vi "Main.vi"() -> ()   [LabVIEW 2017]
doc: "Main Vi para Jogo da Velha Multiplayer - Player x Player na mesma máquina, Player x Player pela rede, Player x Computador"
uses:
  controls/Tabuleiro.ctl
  controls/DataOut.ctl
  controls/GameOption.ctl
  controls/DataIn.ctl
  controls/States.ctl
  controls/LogStates.ctl
  controls/TabuleiroCoordenadas.ctl
panel:
  in  "Reiniciar":bool
  in  "Sair":bool
  out "DataOut":T1
  out "Quem joga":string
  out "Tabuleiro":T2
  # "JOGO DA VELHA"
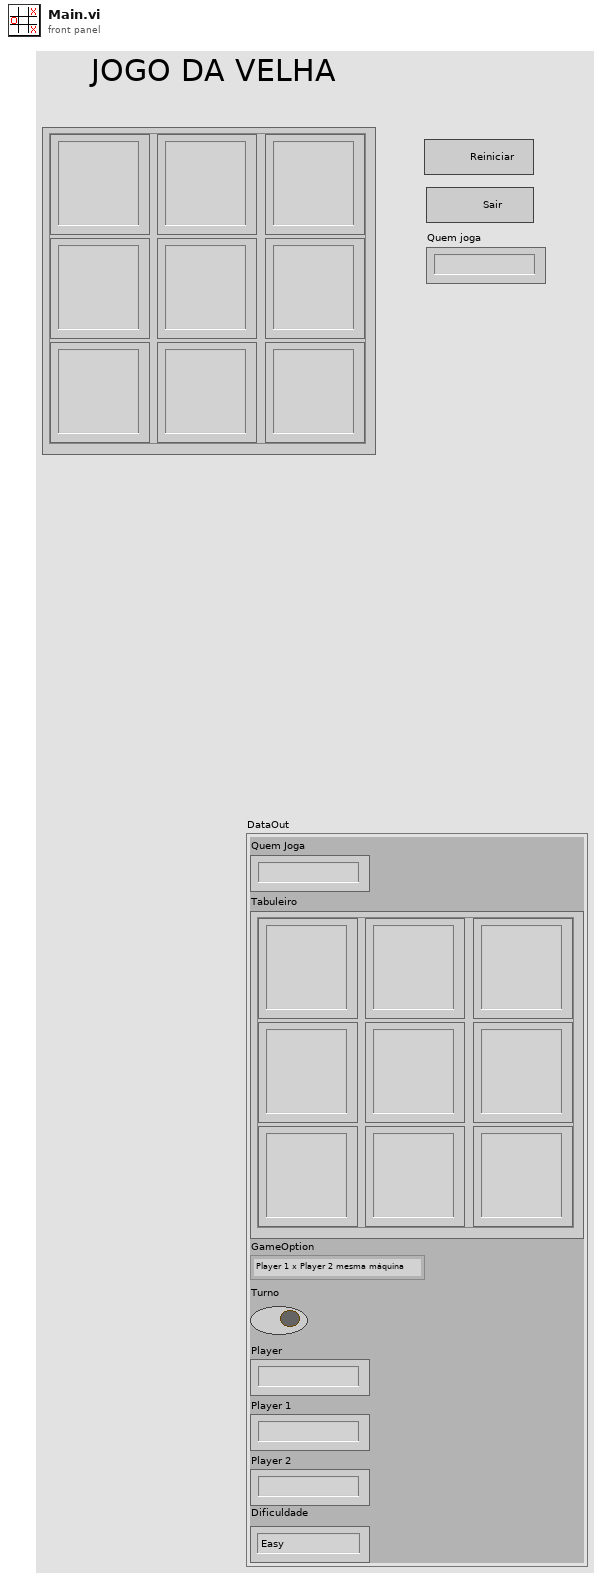
[diagram p1: front panel]
types:
  T1 = typedef "DataOut.ctl" = cluster{"Quem Joga":string, "Tabuleiro":T2, "GameOption":T3, "Turno":bool, "Player":string, "Player 1":string, "Player 2":string, "Dificuldade":enum16{"Easy", "Medium", "Hard"}}
  T2 = typedef "Tabuleiro.ctl" = cluster{"(0,0)":string, "(1,0)":string, "(0,1)":string, "(1,1)":string, "(2,0)":string, "(1,2)":string, "(2,2)":string, "(0,2)":string, "(2,1) ":string}
  T3 = typedef "GameOption.ctl" = enum16{"Player 1 x Player 2 mesma máquina", "Player 1 x Player 2 pela rede", "Player 1 x Computador", "Wait for Event", "Initialize", "Stop"}
  T4 = typedef "States.ctl" = enum16{"Initialize", "Player (wait for event)", "Stop", "PC", "Restart"}
  T5 = typedef "DataIn.ctl" = cluster{"Quem Joga":string, "Tabuleiro":T2, "GameOption":T3, "Turno":bool, "Player":string, "Player 1":string, "Player 2":string, "Dificuldade":enum16{"Easy", "Medium", "Hard"}}
  T6 = typedef "LogStates.ctl" = enum16{"Initialize", "Write", "Write (win, draw)", "Write (PC first)", "Write (Player first)", "Close"}
  T7 = typedef "TabuleiroCoordenadas.ctl" = enum16{"0,0", "0,1", "0,2", "1,0", "1,1", "1,2", "2,0", "2,1", "2,2"}
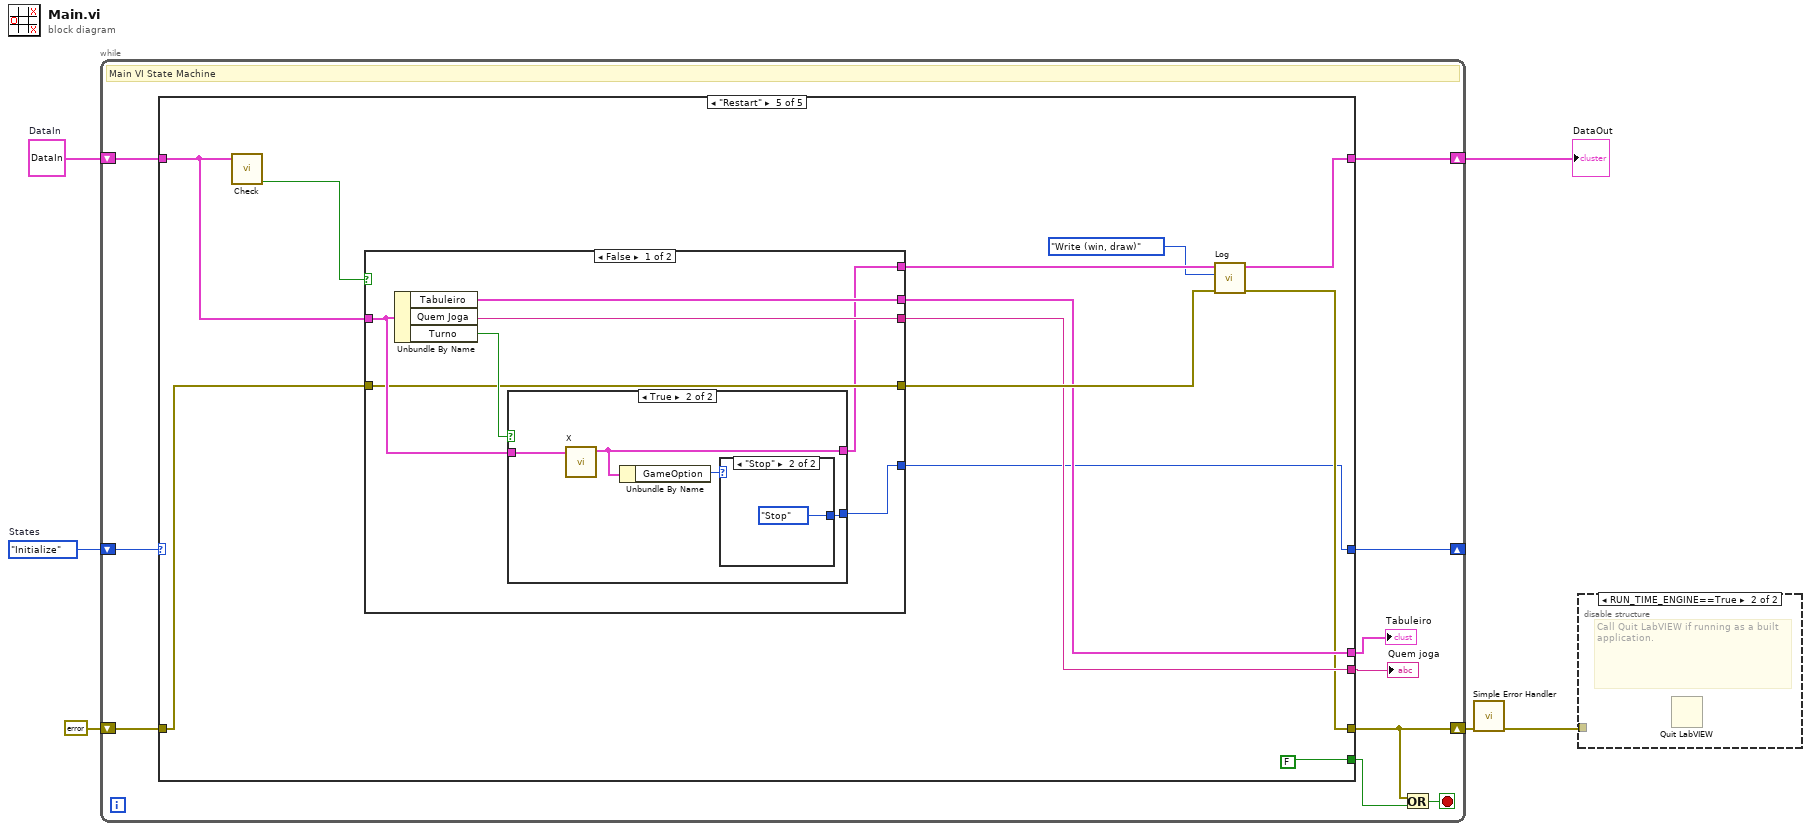
[diagram p0: block diagram]
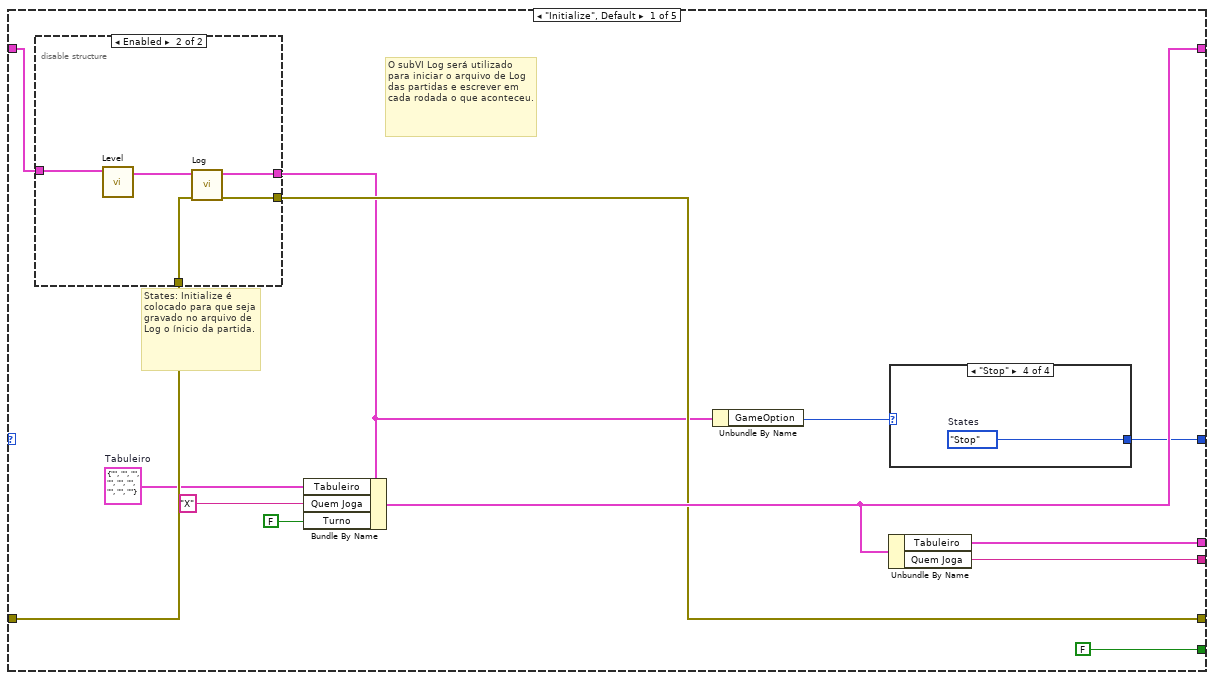
[diagram p2: hidden frame]
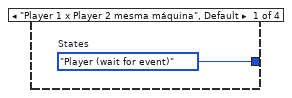
[diagram p3: hidden frame]
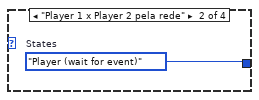
[diagram p4: hidden frame]
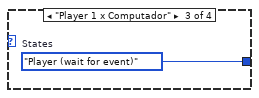
[diagram p5: hidden frame]
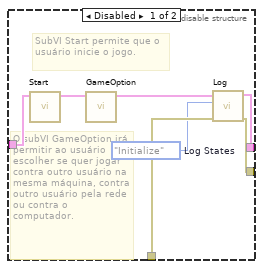
[diagram p6: hidden frame]
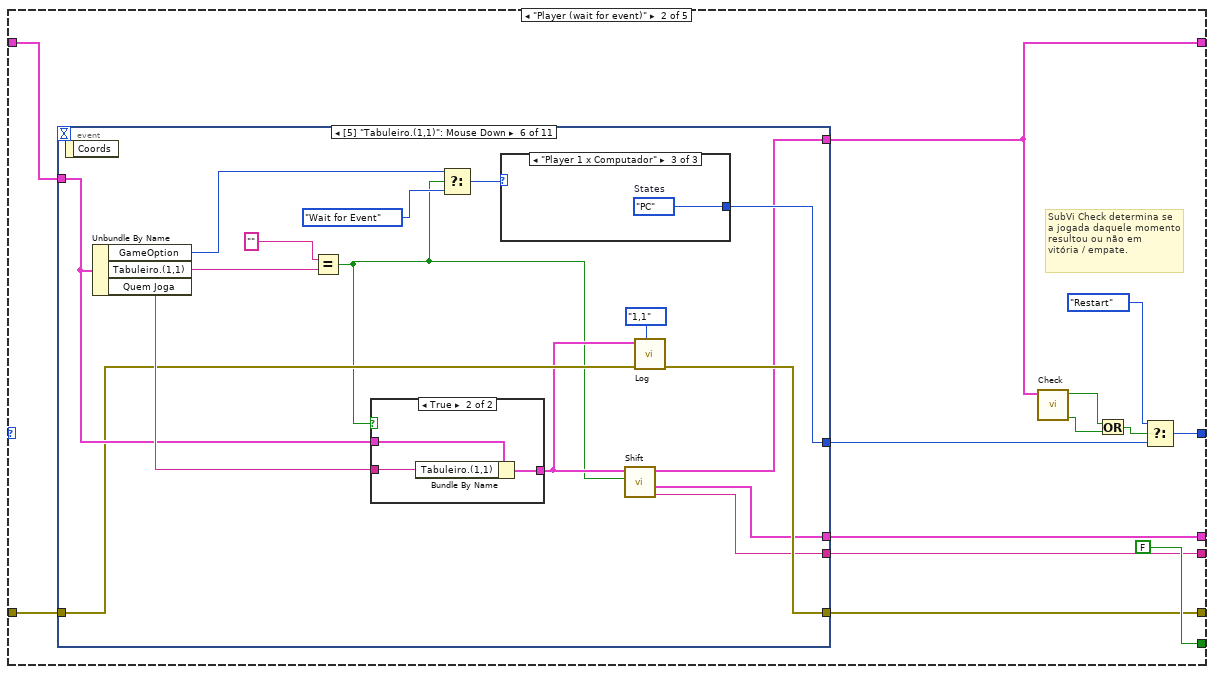
[diagram p7: hidden frame]
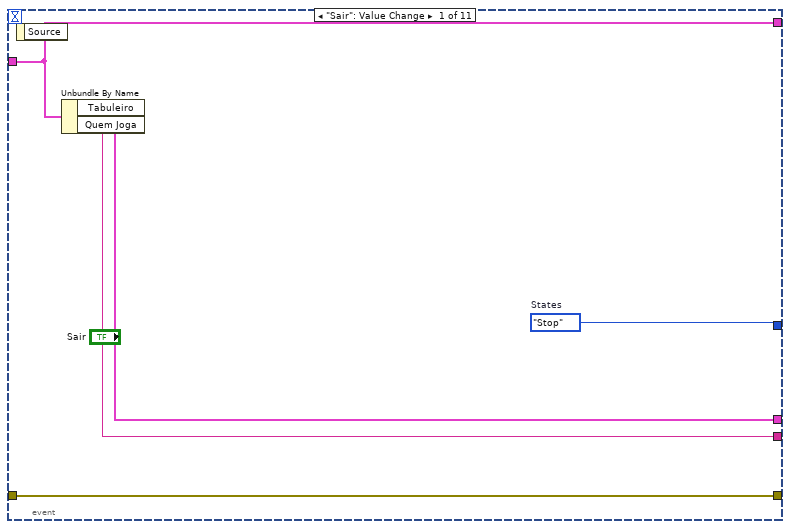
[diagram p8: hidden frame]
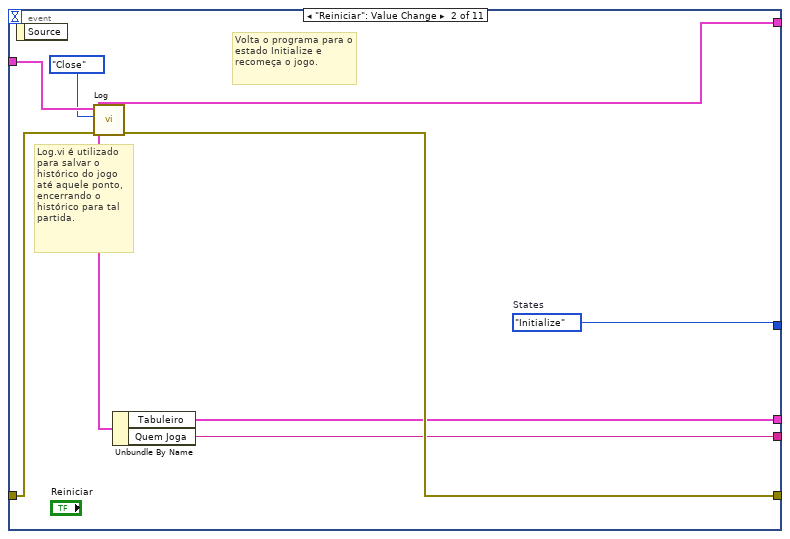
[diagram p9: hidden frame]
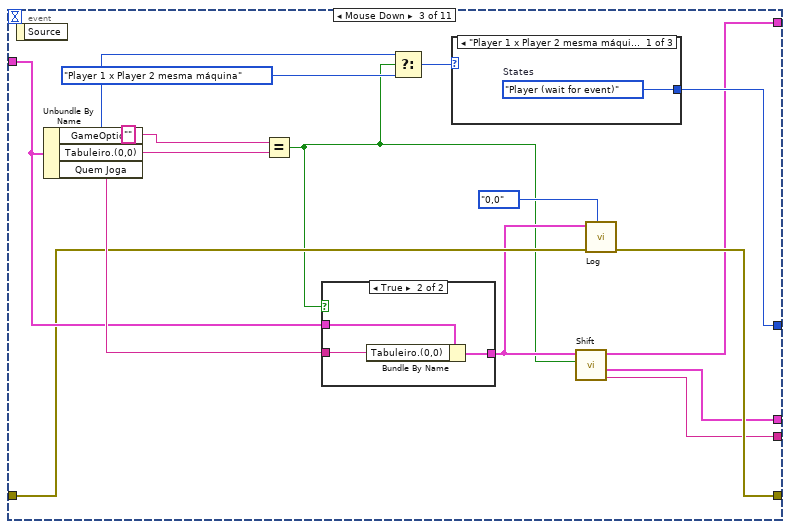
[diagram p10: hidden frame]
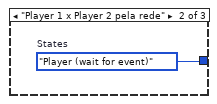
[diagram p12: hidden frame]
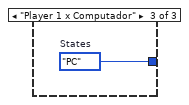
[diagram p13: hidden frame]
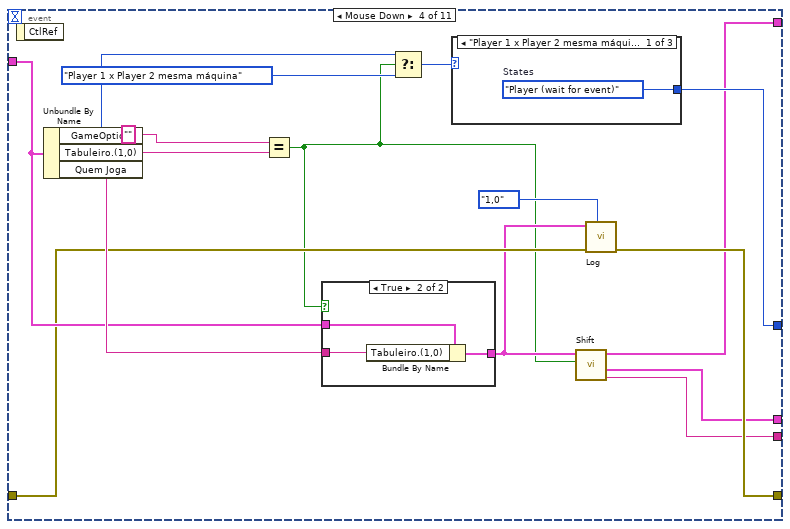
[diagram p14: hidden frame]
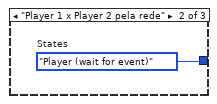
[diagram p16: hidden frame]
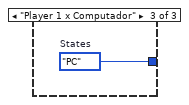
[diagram p17: hidden frame]
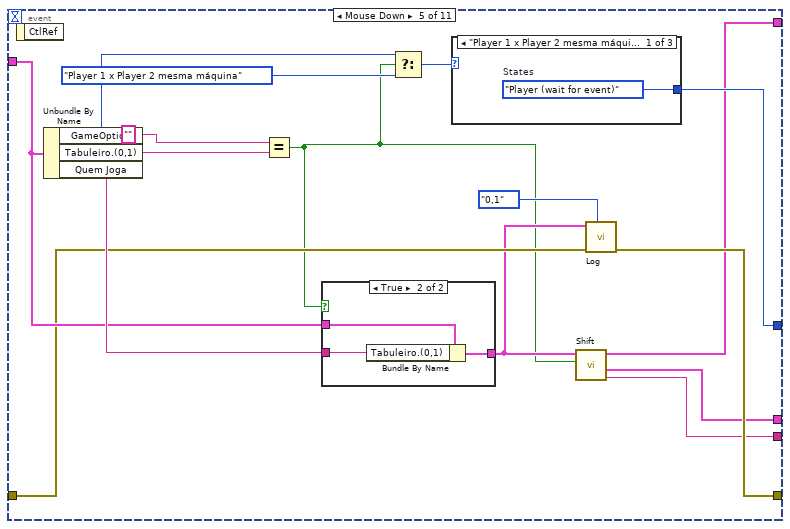
[diagram p18: hidden frame]
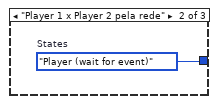
[diagram p20: hidden frame]
diagram:
  w2 = States."Initialize"  # States
  w3 = T5 {"Quem Joga"="", "Tabuleiro"={"(0,0)"="", "(1,0)"="", "(0,1)"="", "(1,1)"="", "(2,0)"="", "(1,2)"="", "(2,2)"="", "(0,2)"="", "(2,1) "=""}, "GameOption"=enum."Player 1 x Player 2 mesma máquina", "Turno"=FALSE, "Player"="", "Player 1"="", "Player 2"="", "Dificuldade"=enum."Easy"}  # DataIn
  n1 = while {
    shift-right: [w13] -> w1
    shift-left: w3 -> [w14]
    shift-right: [w11] -> w5
    shift-left: errorcluster {"status"=FALSE, "code"=0, "source"=""} ("error constant") -> [w12]
    shift-right: [w10] -> _
    shift-left: w2 -> [w15]
    stop <- w16 stop-if-true
    # "Main VI State Machine"
    n2 = case shown="\"Restart\"" w15 {
      tunnel: w14 -> [w28 w57 w282 w286 w313]
      tunnel: [w24 w46 w282 w285 w305] -> w13
      tunnel: w12 -> [w29 w56 w284 w288 w312]
      tunnel: [w20 w55 w284 w288 w306] -> w11
      tunnel: [w17 w51 w283 w291 w304] -> w10
      tunnel: [w23 w54 w281 w290 w310] -> w9
      tunnel: [w22 w53 w280 w289 w309] -> w8
      tunnel: [FALSE FALSE TRUE FALSE FALSE] -> w7
      frame "Initialize", Default {
        w25 = T2 {"(0,0)"="", "(1,0)"="", "(0,1)"="", "(1,1)"="", "(2,0)"="", "(1,2)"="", "(2,2)"="", "(0,2)"="", "(2,1) "=""}  # Tabuleiro
        # "States: Initialize é colocado para que seja gravado no arquivo de Log o ínicio da partida."
        # "O subVI Log será utilizado para iniciar o arquivo de Log das partidas e escrever em cada rodada o que aconteceu."
        n3 = disable-structure shown="Enabled" {
          disable-tunnel: w29 -> [w40 w43]
          disable-tunnel: w28 -> [w39 w41]
          disable-tunnel: [w38 w45] -> w19
          disable-tunnel: [w36 w44] -> w20
          frame Disabled {
            w37 = LogStates."Initialize"  # Log States
            # "SubVI Start permite que o usuário inicie o jogo."
            # "O subVI GameOption irá permitir ao usuário escolher se quer jogar contra outro usuário na mesma máquina, contra outro usuário pela rede ou contra o computador."
            n4 = call "Start.vi"("DataIn"=w39) -> ("Cluster"=w35:T1)  [unwired: 10 in]
            n5 = call "GameOption.vi"("DataIn"=w35) -> ("DataOut"=w34:T1)  [unwired: 10 in]
            n6 = call "Log.vi"("Error In"=w40, "Log States"=w37, "DataIn"=w34) -> ("Error Out"=w36:errorcluster, "DataOut"=w38:T1)  [unwired: 7 in]
          }
          frame Enabled {
            n7 = call "Level.vi"("DataIn"=w41) -> ("Cluster"=w42:T1)  [unwired: 10 in]
            n8 = call "Log.vi"("Error In"=w43, "DataIn"=w42) -> ("Error Out"=w44:errorcluster, "DataOut"=w45:T1)  [unwired: 8 in]
          }
        }
        n9 = Bundle By Name(cluster=w19, "Tabuleiro"=w25, "Quem Joga"="X", "Turno"=FALSE) -> (w24:T1)
        n10 = Unbundle By Name(w19) -> ("GameOption"=w18:T3)
        n11 = Unbundle By Name(w24) -> ("Tabuleiro"=w22:T2, "Quem Joga"=w23:string)
        n12 = case shown="\"Stop\"" w18 {
          tunnel: [w30 w31 w32 w33] -> w17
          frame "Player 1 x Player 2 mesma máquina", Default {
            w30 = States."Player (wait for event)"  # States
          }
          frame "Player 1 x Player 2 pela rede" {
            w31 = States."Player (wait for event)"  # States
          }
          frame "Player 1 x Computador" {
            w32 = States."Player (wait for event)"  # States
          }
          frame "Stop" {
            w33 = States."Stop"  # States
          }
        }
      }
      frame "Player (wait for event)" {
        # "SubVi Check determina se a jogada daquele momento resultou ou não em vitória / empate."
        n13 = event shown="[5] \"Tabuleiro.(1,1)\": Mouse Down" {
          selector: _ -> [_ _ _ _ _ _ _ _ _ _ _]
          dyn-events: _ -> [_ _ _ _ _ _ _ _ _ _ _]
          timeout: _ -> [_ _ _ _ _ _ _ _ _ _ _]
          tunnel: w57 -> [w63 w70 w80 w103 w126 w150 w172 w195 w218 w241 w264]
          tunnel: [w63 w66 w75 w98 w121 w145 w167 w190 w213 w236 w259] -> w46
          tunnel: w56 -> [w62 w68 w78 w101 w124 w148 w170 w193 w216 w239 w262]
          tunnel: [w62 w67 w77 w100 w123 w147 w169 w192 w215 w238 w261] -> w55
          tunnel: [w61 w65 w74 w97 w120 w144 w166 w189 w212 w235 w258] -> w53
          tunnel: [w60 w64 w73 w96 w119 w143 w165 w188 w211 w234 w257] -> w54
          tunnel: [w59 w71 w82 w105 w128 w152 w174 w197 w220 w243 w266] -> w52
          event "Sair": Value Change {
            w59 = States."Stop"  # States
            n14 = event-data() -> ()  [unwired: 1 in, 1 out]
            n15 = Unbundle By Name(w63) -> ("Tabuleiro"=w61:T2, "Quem Joga"=w60:string)
          }
          event "Reiniciar": Value Change {
            w71 = States."Initialize"  # States
            # "Log.vi é utilizado para salvar o histórico do jogo até aquele ponto, encerrando o histórico para tal partida."
            # "Volta o programa para o estado Initialize e recomeça o jogo."
            n16 = event-data() -> ()  [unwired: 1 in, 1 out]
            n17 = call "Log.vi"("Error In"=w68, "Log States"=LogStates."Close", "DataIn"=w70) -> ("Error Out"=w67:errorcluster, "DataOut"=w66:T1)  [unwired: 7 in]
            n18 = Unbundle By Name(w66) -> ("Tabuleiro"=w65:T2, "Quem Joga"=w64:string)
          }
          event Mouse Down {
            n19 = event-data() -> ()  [unwired: 1 in, 1 out]
            n20 = Unbundle By Name(w80) -> ("GameOption"=w84:T3, "Tabuleiro.(0,0)"=w87:string, "Quem Joga"=w81:string)
            n21 = Equal?(x="", y=w87) -> (x = y?=w72:bool)
            n22 = case shown="True" w72 {
              tunnel: w81 -> [_ w90]
              tunnel: w80 -> [w88 w91]
              tunnel: [w88 w89] -> w76
              frame False {
              }
              frame True {
                n23 = Bundle By Name(cluster=w91, "Tabuleiro.(0,0)"=w90) -> (w89:T1)
              }
            }
            n24 = Select(t=w84, s=w72, f=GameOption."Player 1 x Player 2 mesma máquina") -> (s? t:f=w83:T3)
            n25 = case shown="\"Player 1 x Player 2 mesma máquina\", Default" w83 {
              tunnel: [w92 w93 w94] -> w82
              frame "Player 1 x Player 2 mesma máquina", Default {
                w92 = States."Player (wait for event)"  # States
              }
              frame "Player 1 x Player 2 pela rede" {
                w93 = States."Player (wait for event)"  # States
              }
              frame "Player 1 x Computador" {
                w94 = States."PC"  # States
              }
            }
            n26 = call "Shift.vi"("Confirmação"=w72, "DataIn"=w76) -> ("Turno"=w73:string, "Tabuleiro"=w74:T2, "DataOut"=w75:T1)  [unwired: 7 in]
            n27 = call "Log.vi"("Enum Coordenadas"=TabuleiroCoordenadas."0,0" ("Enum"), "Error In"=w78, "DataIn"=w76) -> ("Error Out"=w77:errorcluster)  [unwired: 7 in, 1 out]
          }
          event Mouse Down {
            n28 = event-data() -> ()  [unwired: 1 in, 1 out]
            n29 = Unbundle By Name(w103) -> ("GameOption"=w107:T3, "Tabuleiro.(1,0)"=w110:string, "Quem Joga"=w104:string)
            n30 = Equal?(x="", y=w110) -> (x = y?=w95:bool)
            n31 = case shown="True" w95 {
              tunnel: w104 -> [_ w113]
              tunnel: w103 -> [w111 w114]
              tunnel: [w111 w112] -> w99
              frame False {
              }
              frame True {
                n32 = Bundle By Name(cluster=w114, "Tabuleiro.(1,0)"=w113) -> (w112:T1)
              }
            }
            n33 = Select(t=w107, s=w95, f=GameOption."Player 1 x Player 2 mesma máquina") -> (s? t:f=w106:T3)
            n34 = case shown="\"Player 1 x Player 2 mesma máquina\", Default" w106 {
              tunnel: [w115 w116 w117] -> w105
              frame "Player 1 x Player 2 mesma máquina", Default {
                w115 = States."Player (wait for event)"  # States
              }
              frame "Player 1 x Player 2 pela rede" {
                w116 = States."Player (wait for event)"  # States
              }
              frame "Player 1 x Computador" {
                w117 = States."PC"  # States
              }
            }
            n35 = call "Shift.vi"("Confirmação"=w95, "DataIn"=w99) -> ("Turno"=w96:string, "Tabuleiro"=w97:T2, "DataOut"=w98:T1)  [unwired: 7 in]
            n36 = call "Log.vi"("Enum Coordenadas"=TabuleiroCoordenadas."1,0" ("Enum"), "Error In"=w101, "DataIn"=w99) -> ("Error Out"=w100:errorcluster)  [unwired: 7 in, 1 out]
          }
          event Mouse Down {
            n37 = event-data() -> ()  [unwired: 1 in, 1 out]
            n38 = Unbundle By Name(w126) -> ("GameOption"=w130:T3, "Tabuleiro.(0,1)"=w133:string, "Quem Joga"=w127:string)
            n39 = Equal?(x="", y=w133) -> (x = y?=w118:bool)
            n40 = case shown="True" w118 {
              tunnel: w127 -> [_ w136]
              tunnel: w126 -> [w134 w137]
              tunnel: [w134 w135] -> w122
              frame False {
              }
              frame True {
                n41 = Bundle By Name(cluster=w137, "Tabuleiro.(0,1)"=w136) -> (w135:T1)
              }
            }
            n42 = Select(t=w130, s=w118, f=GameOption."Player 1 x Player 2 mesma máquina") -> (s? t:f=w129:T3)
            n43 = case shown="\"Player 1 x Player 2 mesma máquina\", Default" w129 {
              tunnel: [w138 w139 w140] -> w128
              frame "Player 1 x Player 2 mesma máquina", Default {
                w138 = States."Player (wait for event)"  # States
              }
              frame "Player 1 x Player 2 pela rede" {
                w139 = States."Player (wait for event)"  # States
              }
              frame "Player 1 x Computador" {
                w140 = States."PC"  # States
              }
            }
            n44 = call "Shift.vi"("Confirmação"=w118, "DataIn"=w122) -> ("Turno"=w119:string, "Tabuleiro"=w120:T2, "DataOut"=w121:T1)  [unwired: 7 in]
            n45 = call "Log.vi"("Enum Coordenadas"=TabuleiroCoordenadas."0,1" ("Enum"), "Error In"=w124, "DataIn"=w122) -> ("Error Out"=w123:errorcluster)  [unwired: 7 in, 1 out]
          }
          event Mouse Down {
            n46 = event-data() -> ()  [unwired: 1 in, 1 out]
            n47 = Unbundle By Name(w150) -> ("GameOption"=w141:T3, "Tabuleiro.(1,1)"=w156:string, "Quem Joga"=w151:string)
            n48 = Equal?(x="", y=w156) -> (x = y?=w142:bool)
            n49 = case shown="True" w142 {
              tunnel: w151 -> [_ w159]
              tunnel: w150 -> [w157 w160]
              tunnel: [w157 w158] -> w146
              frame False {
              }
              frame True {
                n50 = Bundle By Name(cluster=w160, "Tabuleiro.(1,1)"=w159) -> (w158:T1)
              }
            }
            n51 = Select(t=w141, s=w142, f=GameOption."Wait for Event") -> (s? t:f=w153:T3)
            n52 = case shown="\"Player 1 x Computador\"" w153 {
              tunnel: [w161 w162 w163] -> w152
              frame "Player 1 x Player 2 mesma máquina", Default {
                w161 = States."Player (wait for event)"  # States
              }
              frame "Player 1 x Player 2 pela rede" {
                w162 = States."Player (wait for event)"  # States
              }
              frame "Player 1 x Computador" {
                w163 = States."PC"  # States
              }
            }
            n53 = call "Shift.vi"("Confirmação"=w142, "DataIn"=w146) -> ("Turno"=w143:string, "Tabuleiro"=w144:T2, "DataOut"=w145:T1)  [unwired: 7 in]
            n54 = call "Log.vi"("Enum Coordenadas"=TabuleiroCoordenadas."1,1" ("Enum"), "Error In"=w148, "DataIn"=w146) -> ("Error Out"=w147:errorcluster)  [unwired: 7 in, 1 out]
          }
          event Mouse Down {
            n55 = event-data() -> ()  [unwired: 1 in, 1 out]
            n56 = Unbundle By Name(w172) -> ("GameOption"=w176:T3, "Tabuleiro.(2,0)"=w179:string, "Quem Joga"=w173:string)
            n57 = Equal?(x="", y=w179) -> (x = y?=w164:bool)
            n58 = case shown="True" w164 {
              tunnel: w173 -> [_ w182]
              tunnel: w172 -> [w180 w183]
              tunnel: [w180 w181] -> w168
              frame False {
              }
              frame True {
                n59 = Bundle By Name(cluster=w183, "Tabuleiro.(2,0)"=w182) -> (w181:T1)
              }
            }
            n60 = Select(t=w176, s=w164, f=GameOption."Player 1 x Player 2 mesma máquina") -> (s? t:f=w175:T3)
            n61 = case shown="\"Player 1 x Player 2 mesma máquina\", Default" w175 {
              tunnel: [w184 w185 w186] -> w174
              frame "Player 1 x Player 2 mesma máquina", Default {
                w184 = States."Player (wait for event)"  # States
              }
              frame "Player 1 x Player 2 pela rede" {
                w185 = States."Player (wait for event)"  # States
              }
              frame "Player 1 x Computador" {
                w186 = States."PC"  # States
              }
            }
            n62 = call "Shift.vi"("Confirmação"=w164, "DataIn"=w168) -> ("Turno"=w165:string, "Tabuleiro"=w166:T2, "DataOut"=w167:T1)  [unwired: 7 in]
            n63 = call "Log.vi"("Enum Coordenadas"=TabuleiroCoordenadas."2,0" ("Enum"), "Error In"=w170, "DataIn"=w168) -> ("Error Out"=w169:errorcluster)  [unwired: 7 in, 1 out]
          }
          event Mouse Down {
            n64 = event-data() -> ()  [unwired: 1 in, 1 out]
            n65 = Unbundle By Name(w195) -> ("GameOption"=w199:T3, "Tabuleiro.(1,2)"=w202:string, "Quem Joga"=w196:string)
            n66 = Equal?(x="", y=w202) -> (x = y?=w187:bool)
            n67 = case shown="True" w187 {
              tunnel: w196 -> [_ w205]
              tunnel: w195 -> [w203 w206]
              tunnel: [w203 w204] -> w191
              frame False {
              }
              frame True {
                n68 = Bundle By Name(cluster=w206, "Tabuleiro.(1,2)"=w205) -> (w204:T1)
              }
            }
            n69 = Select(t=w199, s=w187, f=GameOption."Player 1 x Player 2 mesma máquina") -> (s? t:f=w198:T3)
            n70 = case shown="\"Player 1 x Player 2 mesma máquina\", Default" w198 {
              tunnel: [w207 w208 w209] -> w197
              frame "Player 1 x Player 2 mesma máquina", Default {
                w207 = States."Player (wait for event)"  # States
              }
              frame "Player 1 x Player 2 pela rede" {
                w208 = States."Player (wait for event)"  # States
              }
              frame "Player 1 x Computador" {
                w209 = States."PC"  # States
              }
            }
            n71 = call "Shift.vi"("Confirmação"=w187, "DataIn"=w191) -> ("Turno"=w188:string, "Tabuleiro"=w189:T2, "DataOut"=w190:T1)  [unwired: 7 in]
            n72 = call "Log.vi"("Enum Coordenadas"=TabuleiroCoordenadas."1,2" ("Enum"), "Error In"=w193, "DataIn"=w191) -> ("Error Out"=w192:errorcluster)  [unwired: 7 in, 1 out]
          }
          event Mouse Down {
            n73 = event-data() -> ()  [unwired: 1 in, 1 out]
            n74 = Unbundle By Name(w218) -> ("GameOption"=w222:T3, "Tabuleiro.(2,2)"=w225:string, "Quem Joga"=w219:string)
            n75 = Equal?(x="", y=w225) -> (x = y?=w210:bool)
            n76 = case shown="True" w210 {
              tunnel: w219 -> [_ w228]
              tunnel: w218 -> [w226 w229]
              tunnel: [w226 w227] -> w214
              frame False {
              }
              frame True {
                n77 = Bundle By Name(cluster=w229, "Tabuleiro.(2,2)"=w228) -> (w227:T1)
              }
            }
            n78 = Select(t=w222, s=w210, f=GameOption."Player 1 x Player 2 mesma máquina") -> (s? t:f=w221:T3)
            n79 = case shown="\"Player 1 x Player 2 mesma máquina\", Default" w221 {
              tunnel: [w230 w231 w232] -> w220
              frame "Player 1 x Player 2 mesma máquina", Default {
                w230 = States."Player (wait for event)"  # States
              }
              frame "Player 1 x Player 2 pela rede" {
                w231 = States."Player (wait for event)"  # States
              }
              frame "Player 1 x Computador" {
                w232 = States."PC"  # States
              }
            }
            n80 = call "Shift.vi"("Confirmação"=w210, "DataIn"=w214) -> ("Turno"=w211:string, "Tabuleiro"=w212:T2, "DataOut"=w213:T1)  [unwired: 7 in]
            n81 = call "Log.vi"("Enum Coordenadas"=TabuleiroCoordenadas."2,2" ("Enum"), "Error In"=w216, "DataIn"=w214) -> ("Error Out"=w215:errorcluster)  [unwired: 7 in, 1 out]
          }
          event Mouse Down {
            n82 = event-data() -> ()  [unwired: 1 in, 1 out]
            n83 = Unbundle By Name(w241) -> ("GameOption"=w245:T3, "Tabuleiro.(0,2)"=w248:string, "Quem Joga"=w242:string)
            n84 = Equal?(x="", y=w248) -> (x = y?=w233:bool)
            n85 = case shown="True" w233 {
              tunnel: w242 -> [_ w251]
              tunnel: w241 -> [w249 w252]
              tunnel: [w249 w250] -> w237
              frame False {
              }
              frame True {
                n86 = Bundle By Name(cluster=w252, "Tabuleiro.(0,2)"=w251) -> (w250:T1)
              }
            }
            n87 = Select(t=w245, s=w233, f=GameOption."Player 1 x Player 2 mesma máquina") -> (s? t:f=w244:T3)
            n88 = case shown="\"Player 1 x Player 2 mesma máquina\", Default" w244 {
              tunnel: [w253 w254 w255] -> w243
              frame "Player 1 x Player 2 mesma máquina", Default {
                w253 = States."Player (wait for event)"  # States
              }
              frame "Player 1 x Player 2 pela rede" {
                w254 = States."Player (wait for event)"  # States
              }
              frame "Player 1 x Computador" {
                w255 = States."PC"  # States
              }
            }
            n89 = call "Shift.vi"("Confirmação"=w233, "DataIn"=w237) -> ("Turno"=w234:string, "Tabuleiro"=w235:T2, "DataOut"=w236:T1)  [unwired: 7 in]
            n90 = call "Log.vi"("Enum Coordenadas"=TabuleiroCoordenadas."0,2" ("Enum"), "Error In"=w239, "DataIn"=w237) -> ("Error Out"=w238:errorcluster)  [unwired: 7 in, 1 out]
          }
          event Mouse Down {
            n91 = event-data() -> ()  [unwired: 1 in, 1 out]
            n92 = Unbundle By Name(w264) -> ("GameOption"=w268:T3, "Tabuleiro.(2,1)"=w271:string, "Quem Joga"=w265:string)
            n93 = Equal?(x="", y=w271) -> (x = y?=w256:bool)
            n94 = case shown="True" w256 {
              tunnel: w265 -> [_ w274]
              tunnel: w264 -> [w272 w275]
              tunnel: [w272 w273] -> w260
              frame False {
              }
              frame True {
                n95 = Bundle By Name(cluster=w275, "Tabuleiro.(2,1)"=w274) -> (w273:T1)
              }
            }
            n96 = Select(t=w268, s=w256, f=GameOption."Player 1 x Player 2 mesma máquina") -> (s? t:f=w267:T3)
            n97 = case shown="\"Player 1 x Player 2 mesma máquina\", Default" w267 {
              tunnel: [w276 w277 w278] -> w266
              frame "Player 1 x Player 2 mesma máquina", Default {
                w276 = States."Player (wait for event)"  # States
              }
              frame "Player 1 x Player 2 pela rede" {
                w277 = States."Player (wait for event)"  # States
              }
              frame "Player 1 x Computador" {
                w278 = States."PC"  # States
              }
            }
            n98 = call "Shift.vi"("Confirmação"=w256, "DataIn"=w260) -> ("Turno"=w257:string, "Tabuleiro"=w258:T2, "DataOut"=w259:T1)  [unwired: 7 in]
            n99 = call "Log.vi"("Enum Coordenadas"=TabuleiroCoordenadas."2,1" ("Enum"), "Error In"=w262, "DataIn"=w260) -> ("Error Out"=w261:errorcluster)  [unwired: 7 in, 1 out]
          }
        }
        n100 = call "Check.vi"("DataIn"=w46) -> ("True = Empatou"=w49:bool, "True = Ganhou"=w48:bool)  [unwired: 9 in]
        n101 = Or(x=w48, y=w49) -> (x .or. y?=w47:bool)
        n102 = Select(t=States."Restart", s=w47, f=w52) -> (s? t:f=w51:T4)
      }
      frame "Stop" {
        w283 = States."Stop"  # States
        n103 = Unbundle By Name(w282) -> ("Tabuleiro"=w280:T2, "Quem Joga"=w281:string)
      }
      frame "PC" {
        w292 = States."Player (wait for event)"  # States
        w293 = States."Restart"  # States
        # "True - Médio\nFalse - Fácil"
        # "Caso a jogada tenha resultado em vitória ou empate, encaminha o programa para o estado Restart. Caso ainda não exista vencedor, nem tenha ocorrido um empate, encaminha o programa para o estado wait for event para a próxima jogada."
        # "SubVI Check confere se a jogada culminou em vitória ou empate."
        n104 = Unbundle By Name(w286) -> ("Dificuldade"=w287:enum16{"Easy", "Medium", "Hard"})
        n105 = case shown="\"Hard\"" w287 {
          tunnel: w286 -> [w298 w301 w302]
          tunnel: [w299 w300 w303] -> w285
          frame "Easy", Default {
            n106 = call "SimpleMove.vi"("DataIn"=w298) -> ("DataOut"=w299:T1)  [unwired: 10 in]
          }
          frame "Medium" {
            n107 = call "PC.vi"("DataIn"=w301) -> ("DataOut"=w300:T1)  [unwired: 10 in]
          }
          frame "Hard" {
            n108 = call "PC Hard.vi"("DataIn"=w302) -> ("DataOut"=w303:T1)  [unwired: 10 in]
          }
        }
        n109 = call "Check.vi"("DataIn"=w285) -> ("True = Empatou"=w295:bool, "True = Ganhou"=w296:bool)  [unwired: 9 in]
        n110 = Unbundle By Name(w285) -> ("Tabuleiro"=w289:T2, "Quem Joga"=w290:string)
        n111 = Or(x=w296, y=w295) -> (x .or. y?=w294:bool)
        n112 = Select(t=w293, s=w294, f=w292) -> (s? t:f=w291:T4)
      }
      frame "Restart" {
        n113 = call "Check.vi"("DataIn"=w313) -> ("True = Empatou"=w314:bool)  [unwired: 9 in, 1 out]
        n114 = case shown="False" w314 {
          tunnel: w313 -> [w319 w341]
          tunnel: w312 -> [w318 w340]
          tunnel: [w318 w340] -> w311
          tunnel: [w321 w339] -> w309
          tunnel: [w320 w338] -> w310
          tunnel: [w317 w337] -> w308
          tunnel: [w316 w335] -> w304
          frame False {
            n115 = Unbundle By Name(w319) -> ("Tabuleiro"=w321:T2, "Quem Joga"=w320:string, "Turno"=w322:bool)
            n116 = case shown="True" w322 {
              tunnel: w319 -> [w326 w332]
              tunnel: [w325 w331] -> w317
              tunnel: [w323 w329] -> w316
              frame False {
                n117 = call "O.vi"("DataIn"=w326) -> ("DataOut"=w325:T1)  [unwired: 10 in]
                n118 = Unbundle By Name(w325) -> ("GameOption"=w324:T3)
                n119 = case shown="\"Stop\"" w324 {
                  tunnel: [States."Stop" ("States") States."Initialize" ("States")] -> w323
                  frame "Stop" {
                  }
                  frame "Initialize", Default {
                  }
                }
              }
              frame True {
                n120 = call "X.vi"("DataIn"=w332) -> ("DataOut"=w331:T1)  [unwired: 10 in]
                n121 = Unbundle By Name(w331) -> ("GameOption"=w330:T3)
                n122 = case shown="\"Stop\"" w330 {
                  tunnel: [States."Initialize" ("States") States."Stop" ("States")] -> w329
                  frame "Initialize", Default {
                  }
                  frame "Stop" {
                  }
                }
              }
            }
          }
          frame True {
            n123 = call "Draw.vi"("DataIn"=w341) -> ("DataOut"=w337:T1)  [unwired: 10 in]
            n124 = Unbundle By Name(w337) -> ("Tabuleiro"=w339:T2, "Quem Joga"=w338:string, "GameOption"=w336:T3)
            n125 = case shown="\"Initialize\", Default" w336 {
              tunnel: [w342 States."Stop" ("States")] -> w335
              frame "Initialize", Default {
                w342 = States."Initialize"  # States
              }
              frame "Stop" {
              }
            }
          }
        }
        n126 = call "Log.vi"("Error In"=w311, "Log States"=LogStates."Write (win, draw)", "DataIn"=w308) -> ("Error Out"=w306:errorcluster, "DataOut"=w305:T1)  [unwired: 7 in]
      }
    }
    "Quem joga" <- w9
    "Tabuleiro" <- w8
    n127 = Or(x=w11, y=w7) -> (x .or. y?=w16:bool)
  }
  "DataOut" <- w1
  n128 = call <vilib>:"Simple Error Handler.vi"("error in (no error)"=w5) -> ("error out"=w4:errorcluster)  [unwired: 4 in, 4 out]
  n129 = disable-structure shown="RUN_TIME_ENGINE==True" {
    disable-tunnel: w4 -> [_ _]
    frame condition #0 (active) {
    }
    frame condition #1 {
      # "Call Quit LabVIEW if running as a built application."
      n130 = Quit LabVIEW() -> ()  [unwired: 1 in]
    }
  }
